vi "Read JSON Config.vi"(8 "error in (no error)":errorcluster, 10 "JSON Config":string, 11 "abs_SharedVar_Bool in":refnum<class "conc_SharedVar_I32.lvclass">) -> (0 "error out":errorcluster, 3 "abs_SharedVar_Bool out":refnum<class "conc_SharedVar_I32.lvclass">)   [LabVIEW 2021, in "conc_SharedVar_I32.lvclass"]
uses:
  conc_SharedVar_I32.lvclass
  C:/Program Files (x86)/National Instruments/LabVIEW 2021/vi.lib/TSA/Abstract Data Classes/Abs_Types/Type/Abs_Type.lvclass
  conc_SharedVar_I32.lvclass/conc_SharedVar_I32.ctl
  c4a07f48-c01b-4824-9756-c00d686fd904.vi
  <vilib>/JDP Science/JSONtext/Find Item.vi
  <vilib>/JDP Science/JSONtext/Next JSON Value.vi
  <vilib>/JDP Science/JSONtext/String Subset.vi
  <vilib>/JDP Science/JSONtext/Parsing/Advance past next JSON Value (inlined COPY).vi
  <vilib>/JDP Science/JSONtext/Parsing/Advance past whitespace.vi
  <vilib>/JDP Science/JSONtext/Parsing/Advance past String.vi
  <vilib>/JDP Science/JSONtext/Parsing/Advance past Number.vi
  <vilib>/JDP Science/JSONtext/Parsing/Advance past Line Ending.vi
  <vilib>/Utility/LVClass/Get LV Class Name.vi
  <vilib>/JDP Science/JSONtext/Parsing/Parse Full Path or Item Name.vi
  <vilib>/JDP Science/JSONtext/Parsing/Advance past Array.vi
  <vilib>/JDP Science/JSONtext/Parsing/Advance past Object.vi
  <vilib>/JDP Science/JSONtext/support/Error Cluster From Code.vi
  <vilib>/JDP Science/JSONtext/Offset/Find Item Locations by Path.vi
  <vilib>/JDP Science/JSONtext/JSON text to Variant.vi
  <vilib>/JDP Science/JSONtext/LVClass Serializer/JSONtext LVClass Serializer.lvclass
  <vilib>/TSA/Abstract Data Classes/Abs_Types/I32 Integer/Abs_I32 Integer.lvclass
  <vilib>/TSA/Abstract Data Classes/Abs_Types/Type/Abs_Type.lvclass
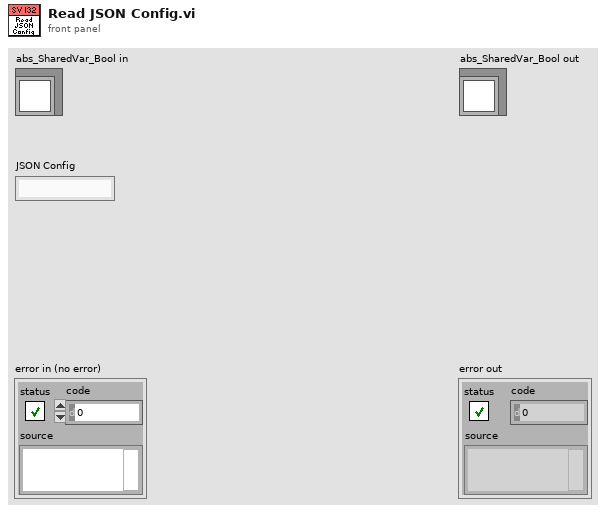
[diagram p1: front panel]
types:
  T1 = cluster{"Shared Variable Refnum":refnum<k21>, "Write Access":enum8{"Allowed", "Required", "None"}, "Read Access":enum8{"Allowed", "Required", "None"}}
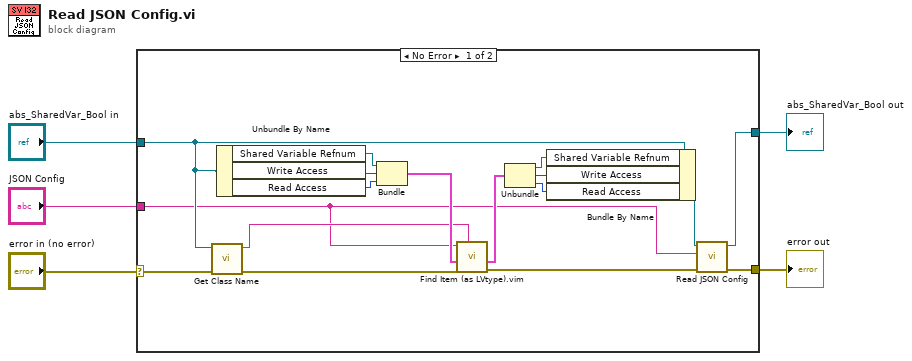
[diagram p0: block diagram]
diagram:
  n1 = case shown="No Error" "error in (no error)" {
    selector: "error in (no error)" -> [w18 w23]
    tunnel: [w22 w23] -> w5
    tunnel: [w21 w24] -> w4
    tunnel: "JSON Config" -> [w6 _]
    tunnel: "abs_SharedVar_Bool in" -> [w13 w24]
    frame No Error {
      n2 = call <vilib>:"Get Class Name.vi"("error in (no error)"=w18, "Abs_Type in"=w13) -> ("error out"=w19:errorcluster, "class name"=w10:string)  [unwired: 8 in]
      n3 = Unbundle By Name(w13) -> ("Shared Variable Refnum"=w17:refnum<k21>, "Write Access"=w16:enum8{"Allowed", "Required", "None"}, "Read Access"=w15:enum8{"Allowed", "Required", "None"})
      n4 = Bundle("Shared Variable Refnum"=w17, "Write Access"=w16, "Read Access"=w15) -> (w14:T1)  [unwired: 1 in]
      n5 = call "Find Item (as LVtype).vim"("$Path or Item Name"=w10, "error in (no error)"=w19, "Data Type and Default Value"=w14, "JSON"=w6) -> ("error out"=w20:errorcluster, "Data"=w12:T1)  [unwired: 4 in, 2 out]
      n6 = Unbundle(w12) -> ("Shared Variable Refnum"=w9:refnum<k21>, "Write Access"=w8:enum8{"Allowed", "Required", "None"}, "Read Access"=w7:enum8{"Allowed", "Required", "None"})
      n7 = Bundle By Name(cluster=w13, "Shared Variable Refnum"=w9, "Write Access"=w8, "Read Access"=w7) -> (w11:refnum<class "conc_SharedVar_I32.lvclass">)
      n8 = call-parent "Read JSON Config.vi"("error in (no error)"=w20, "JSON Config"=w6, "Abs_Type in"=w11) -> ("error out"=w22:errorcluster, "Abs_Type out"=w21:refnum<class "conc_SharedVar_I32.lvclass">)  [unwired: 7 in]
    }
    frame Error {
    }
  }
  "error out" <- w5
  "abs_SharedVar_Bool out" <- w4
